vi "Instrument Type ID.vi"() -> (1 "instrument type id":string="comVISA")   [LabVIEW 2020, in "VISA Measurement.lvlib"]
uses:
  VISA Measurement.lvlib
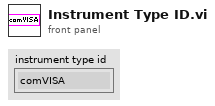
[diagram p1: front panel]
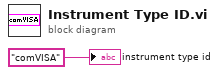
[diagram p0: block diagram]
diagram:
  "instrument type id" <- "comVISA"
